vi "Update Output Latch.vi"   [LabVIEW 2014, in "SLSC configuration Shared.lvlib"]
doc: "Update the output latch of the pins."
uses:
  SLSC configuration Shared.lvlib
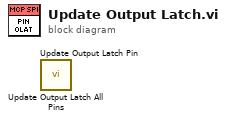
[diagram p0: block diagram]
diagram:
  n1 = call "Update Output Latch All Pins.vi"() -> ()  [unwired: 9 in, 3 out]
  n2 = call "Update Output Latch Pin.vi"() -> ()  [unwired: 9 in, 3 out]
